vi "Upper Left.vi"(0 "VI in":refnum<vi>, 3 "error in":errorcluster, 4 "FP.WinBounds In":T1) -> (6 "FP.WinBounds Out":T1, 7 "ref out":refnum<vi>, 10 "error out":errorcluster)   [LabVIEW 2014]
doc: "Upper Left\n\nSets BAE6's front panel onto the upper left corner of the monitor.\n\nBeverly Abadines\nPHY 350\nE6"
uses:
  <vilib>/Utility/miscctls.llb/LVRectTypeDef.ctl
panel:
  # "Upper Left"
  # "Beverly Abadines\nPhys 350\nE6"
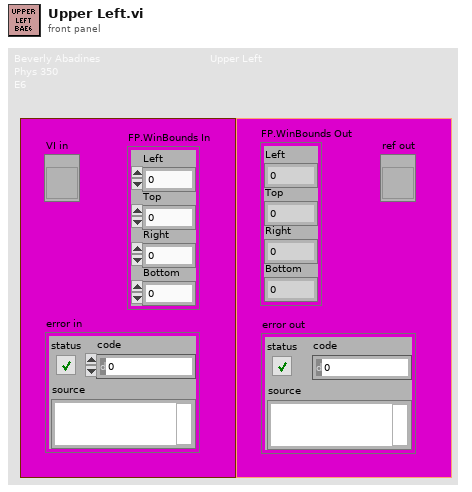
[diagram p1: front panel]
types:
  T1 = typedef "LVRectTypeDef.ctl" = cluster{"Left":i16, "Top":i16, "Right":i16, "Bottom":i16}
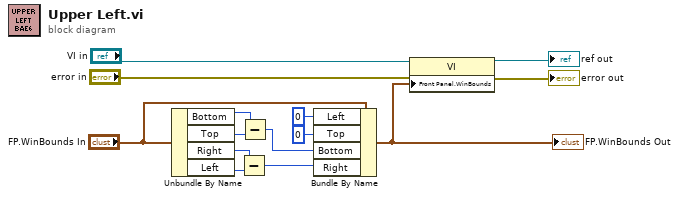
[diagram p0: block diagram]
diagram:
  n1 = Unbundle By Name("FP.WinBounds In") -> ("Bottom"=w10:i16, "Top"=w11:i16, "Right"=w7:i16, "Left"=w8:i16)
  n2 = Subtract(x=w7, y=w8) -> (x-y=w6:i16)
  n3 = Subtract(x=w10, y=w11) -> (x-y=w9:i16)
  n4 = Bundle By Name(cluster="FP.WinBounds In", "Left"=i16 0, "Top"=i16 0, "Bottom"=w9, "Right"=w6) -> (w1:T1)
  "FP.WinBounds Out" <- w1
  n5 = property class="VI"(reference="VI in", error in="error in", "Front Panel.WinBounds"=w1) -> (reference out=→"ref out":refnum<vi>, error out=→"error out":errorcluster)
